vi "Serve Team Data.vi"(11 "LabVIEW Web Service Request":refnum<class "Web Request.lvclass">) -> ()   [LabVIEW 2013]
uses:
  <vilib>/wsapi/Web Request.lvclass
  <vilib>/xml/Close Reference(Node).vi
  <vilib>/xml/NI_XML.lvlib
  <resource>/objmgr/DOMUserDefRef.rc
panel:
  out "XML":string
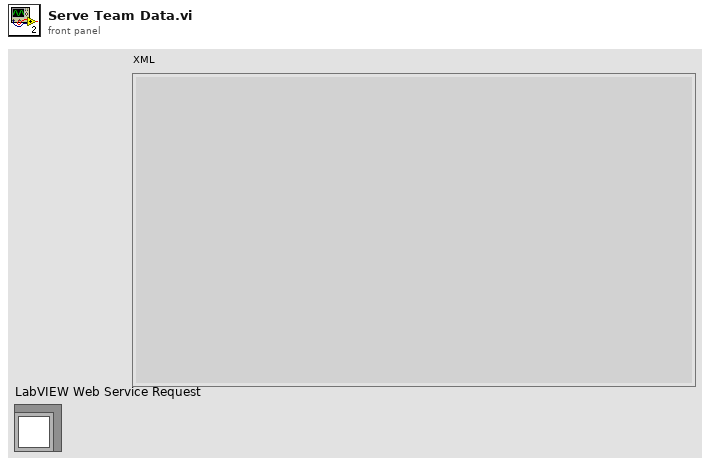
[diagram p1: front panel]
types:
  T1 = enum16{"Get Teams", "Add Team", "Modify Team", "Clear All Teams"}
  T2 = typedef "Team Data.ctl" = cluster{"Both":string, "Name":string, "GUID":u16, "Number":u16}
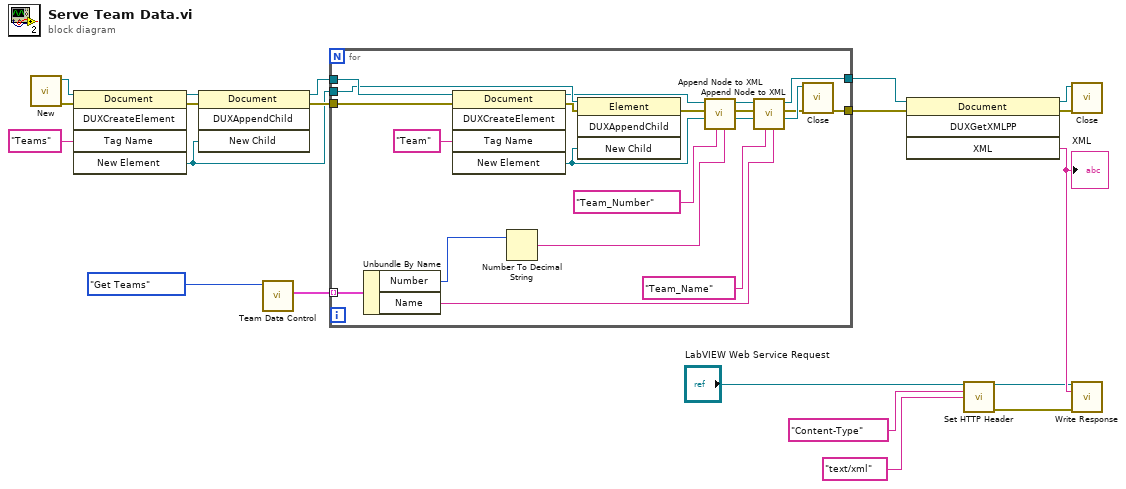
[diagram p0: block diagram]
diagram:
  n1 = call <vilib>:"New.vi"() -> ("error out"=w19:errorcluster, "DOM document out"=w20:refnum<k20>)  [unwired: 8 in]
  n2 = invoke class="Document" method="DUXCreateElement"(reference=w20, error in=w19, "Tag Name"="Teams") -> (reference out=w17:refnum<k20>, error out=w16:errorcluster, "New Element"=w13:refnum<k20>)  [unwired: 2 in, 2 out]
  n3 = invoke class="Document" method="DUXAppendChild"(reference=w17, error in=w16, "New Child"=w13) -> (reference out=w15:refnum<k20>, error out=w14:errorcluster)  [unwired: 1 in, 2 out]
  n4 = call "Team Data Control.vi"("Mode"=T1."Get Teams") -> ("Team Array Out"=w6:T2[])  [unwired: 10 in]
  n5 = for {
    tunnel: w6 -> [w34] mode=indexing
    tunnel: w15 -> [w41]
    tunnel: w14 -> [w40]
    tunnel: w13 -> [w38]
    tunnel: [w31] -> w12
    tunnel: [w28] -> w11
    n6 = Unbundle By Name(w34) -> ("Number"=w27:u16, "Name"=w22:string)
    n7 = invoke class="Document" method="DUXCreateElement"(reference=w41, error in=w40, "Tag Name"="Team") -> (reference out=w36:refnum<k20>, error out=w37:errorcluster, "New Element"=w26:refnum<k20>)  [unwired: 2 in, 2 out]
    n8 = Number To Decimal String(number=w27) -> (decimal integer string=w25:string)  [unwired: 1 in]
    n9 = invoke class="Element" method="DUXAppendChild"(reference=w38, error in=w37, "New Child"=w26) -> (error out=w35:errorcluster)  [unwired: 1 in, 3 out]
    n10 = call "Append Node to XML.vi"("Data"=w25, "Tag Name"="Team_Number", "SuperElement In"=w26, "error in"=w35, "DOM document in"=w36) -> ("SuperElement Out"=w23:refnum<k20>, "error out"=w32:errorcluster, "DOM document out"=w33:refnum<k20>)  [unwired: 4 in]
    n11 = call "Append Node to XML.vi"("Data"=w22, "Tag Name"="Team_Name", "SuperElement In"=w23, "error in"=w32, "DOM document in"=w33) -> ("SuperElement Out"=w30:refnum<k20>, "error out"=w29:errorcluster, "DOM document out"=w31:refnum<k20>)  [unwired: 4 in]
    n12 = call-poly <vilib>:"Close.vi"("error in (no error)"=w29, "node"=w30) -> ("error out"=w28:errorcluster)  [unwired: 7 in]
  }
  n13 = invoke class="Document" method="DUXGetXMLPP"(reference=w12, error in=w11) -> (reference out=w10:refnum<k20>, error out=w9:errorcluster, "XML"=w8:string)  [unwired: 2 in, 1 out]
  "XML" <- w8
  n14 = call <vilib>:"Set HTTP Header.vi"("LabVIEW Web Service Request"="LabVIEW Web Service Request", "header"="Content-Type", "header value"="text/xml") -> ("LabVIEW Web Service Request out"=w2:refnum<class "Web Request.lvclass">, "error out"=w1:errorcluster)  [unwired: 11 in]
  n15 = call-poly <vilib>:"Close.vi"("error in (no error)"=w9, "node"=w10) -> ()  [unwired: 7 in, 1 out]
  n16 = call <vilib>:"Write Response.vi"("LabVIEW Web Service Request"=w2, "response string"=w8, "error in (no error)"=w1) -> ()  [unwired: 11 in, 2 out]
